vi "波形图表刷新模式.vi"() -> ()   [LabVIEW 2010]
uses:
  <vilib>/Analysis/NI_AALBase.lvlib
panel:
  out "波形图表 3":dbl[](graph)
  out "波形图表 2":dbl[](graph)
  out "波形图表":dbl[](graph)
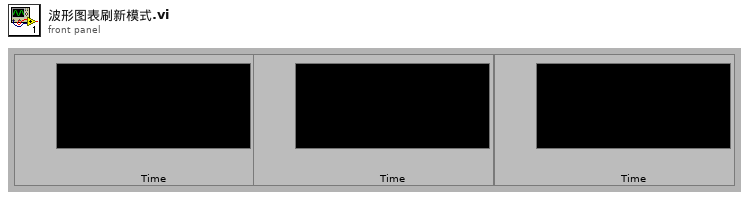
[diagram p1: front panel]
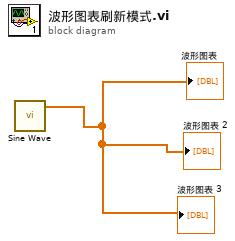
[diagram p0: block diagram]
diagram:
  n1 = call <vilib>:"Sine Wave.vi"() -> ("sine wave"=→"波形图表" →"波形图表 2" →"波形图表 3":dbl[])  [unwired: 5 in, 2 out]
